vi "CALC_OFFS_PHAS.vi"(0 "VISA IN":refnum<visa-resource-name>, 1 "Offset Phase Value":i32, 2 "Units for Phase":string(combo)="DEG", 5 "error in":errorcluster, 7 "Channel":i32=1) -> (14 "VISA Out":refnum<visa-resource-name>, 19 "error out":errorcluster)   [LabVIEW 2018, in "PNA-X.lvlib"]
doc: "CALCulate<cnum>:OFFSet:PHASe <num>[<char>] \n1551\n\n(Read-Write) Sets the phase offset for the selected measurement. \nSee Critical Note \nParameters \n<cnum> Channel number of the measurement. There must be a selected measurement \non that channel. If unspecified, <cnum> is set to 1. \n<num> Offset phase value. Choose any number between: \n-360 and 360 \n<char> Units for phase. OPTIONAL. Choose either: \nDEG - Degrees (default) \nRAD - Radians \nExamples CALC:OFFS:PHAS 10 \ncalculate:offset:phase 20rad \nQuery Syntax CALCulate:OFFSet:PHASe? \nReturn Type Numeric, returned value always in degrees \nDefault 0 degrees \n1552\n\nCalculate:Parameter Commands \nLists, creates, selects and deletes measurements. \nClick on a blue keyword to view the command details. \nSee Also \nExample Programs \nLearn about Measurement Parameters \nSynchronizing the PNA and Controller \nSCPI Command Tree \nCritical Note: CALCulate commands act on the selected measurement. You can select one \nmeasurement for each channel using Calc:Par:Select"
uses:
  PNA-X.lvlib
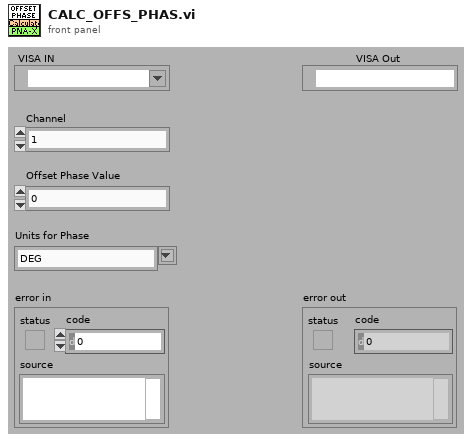
[diagram p1: front panel]
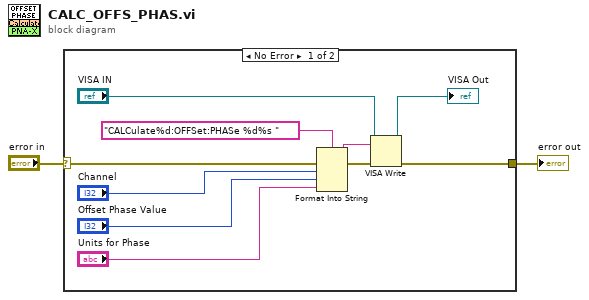
[diagram p0: block diagram]
diagram:
  n1 = case shown="No Error" "error in" {
    selector: "error in" -> [w12 w13]
    tunnel: [w7 w13] -> w1
    frame No Error {
      n2 = Format Into String(format string="CALCulate%d:OFFSet:PHASe %d%s " ("Cmdline"), error in=w12, "Channel", "Offset Phase Value", "Units for Phase") -> (resulting string=w10:string, error out=w11:errorcluster)  [unwired: 1 in]
      n3 = VISA Write(VISA resource name="VISA IN", write buffer=w10, error in (no error)=w11) -> (VISA resource name out=→"VISA Out":refnum<visa-resource-name>, error out=w7:errorcluster)  [unwired: 1 out]
    }
    frame Error {
    }
  }
  "error out" <- w1
